vi "NegativeExponentialSampleTrain.vi"(10 "Sample rate":i32, 11 "Time (ms)":i32) -> (2 "ImpulseTrain":dbl[](array[numeric]))   [LabVIEW 2023]
doc: "Generates an impulse train of a given time in ms."
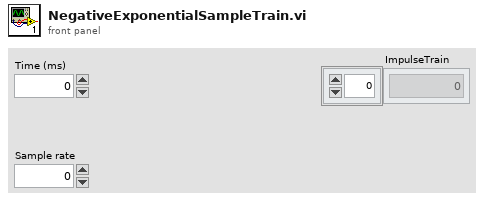
[diagram p1: front panel]
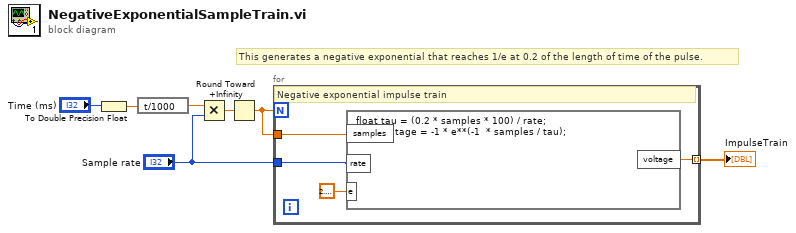
[diagram p0: block diagram]
diagram:
  # "This generates a negative exponential that reaches 1/e at 0.2 of the length of time of the pulse."
  n1 = To Double Precision Float(number="Time (ms)") -> (double precision float=w3:dbl)
  n2 = expression code="t/1000"(w3) -> (w5:dbl)
  n3 = Multiply(x=w5, y="Sample rate") -> (x*y=w2:dbl)
  n4 = Round Toward +Infinity(x=w2) -> (ceil(x): smallest int >= x=w1:dbl)
  n5 = for {
    N: w1 -> [_]
    tunnel: w1 -> [w8]
    tunnel: "Sample rate" -> [w11]
    tunnel: [w10] -> w7 mode=indexing
    # "Negative exponential impulse train"
    n6 = formula code="float tau = (0.2 * samples * 100) / rate;\nfloat voltage = -1 * e**(-1  * samples / tau);"("samples"=w8, "rate"=w11, "e"=2.718281828459045) -> ("voltage"=w10:dbl)
  }
  "ImpulseTrain" <- w7
